vi "Set ADC.vi"(8 "error in (no error)":errorcluster, 10 "Configure ADS1115":T1={"Mode"=enum."Single-Shot", "MUX"=enum."Single AI3 - GND", "Data Rate"=enum."8 SPS", "PGA"=enum."FS = ±6.144V"}, 11 "ADS1115 in":refnum<class "Grove An In ADS1115.lvclass">) -> (0 "error out":errorcluster, 3 "ADS1115 out":refnum<class "Grove An In ADS1115.lvclass">)   [LabVIEW 2020, in "CTI-Peripheral.lvlib" / "Grove An In ADS1115.lvclass"]
uses:
  Grove An In ADS1115.lvclass
  Private/ConfigData.ctl
  Private/ADS1115Mode.ctl
  Private/ADS1115Mux.ctl
  Private/ADS1115DataRate.ctl
  Private/ADS1115PGA.ctl
  Grove An In ADS1115.lvclass/Grove An In ADS1115.ctl
  CTI/I2C Connection/I2C Connection.lvclass/I2C Connection.ctl
  CTI/Session/I2C Write Data.vi
  CTI/Session/I2C Read Data.vi
  CTI/I2C Connection/I2C Connection.lvclass
panel:
  out "Data":string
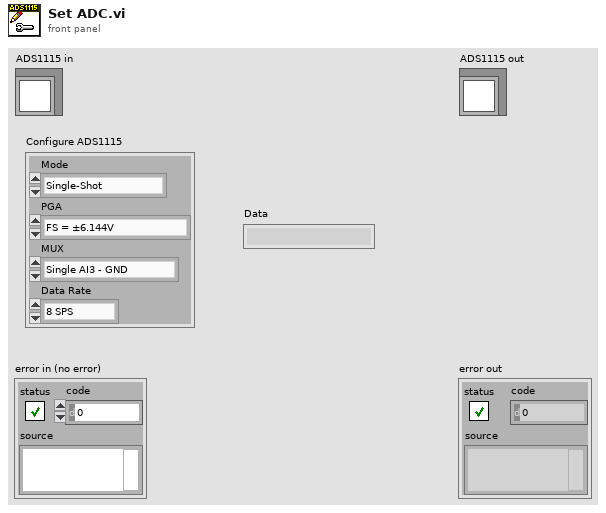
[diagram p1: front panel]
types:
  T1 = typedef "ConfigData.ctl" = cluster{"Mode":T2, "MUX":T3, "Data Rate":T4, "PGA":T5}
  T2 = typedef "CTI-Peripheral.lvlib/Grove An In ADS1115.lvclass/ADS1115Mode.ctl" = enum16{"Continuous", "Single-Shot"}
  T3 = typedef "CTI-Peripheral.lvlib/Grove An In ADS1115.lvclass/ADS1115Mux.ctl" = enum16{"Single AI0 - GND", "Single AI1 - GND", "Single AI2 - GND", "Single AI3 - GND"}
  T4 = typedef "CTI-Peripheral.lvlib/Grove An In ADS1115.lvclass/ADS1115DataRate.ctl" = enum16{"8 SPS", "16 SPS", "32 SPS", "64 SPS", "128 SPS", "250 SPS", "475 SPS", "860 SPS"}
  T5 = typedef "CTI-Peripheral.lvlib/Grove An In ADS1115.lvclass/ADS1115PGA.ctl" = enum16{"FS = ±6.144V", "FS = ±4.096V", "FS = ±2.048V", "FS = ±1.024V", "FS = ±0.512V", "FS = ±0.256V"}
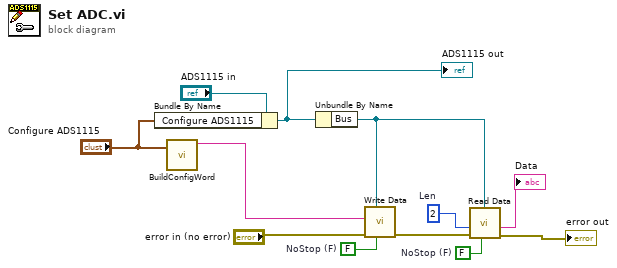
[diagram p0: block diagram]
diagram:
  w9 = FALSE  # NoStop (F)
  w10 = u8 2  # Len
  w11 = FALSE  # NoStop (F)
  n1 = Bundle By Name(cluster="ADS1115 in", "Configure ADS1115"="Configure ADS1115") -> (w1:refnum<class "Grove An In ADS1115.lvclass">)
  "ADS1115 out" <- w1
  n2 = call "BuildConfigWord.vi"("NewVal"="Configure ADS1115") -> ("string"=w5:string)  [unwired: 10 in]
  n3 = Unbundle By Name(w1) -> ("Bus"=w8:refnum<class "I2C Connection.lvclass">)
  n4 = call "Write Data.vi"("NoStop (F)"=w11, "I2C Connection"=w8, "error in (no error)"="error in (no error)", "Data"=w5) -> ("error out"=w7:errorcluster)  [unwired: 7 in]
  n5 = call "Read Data.vi"("NoStop (F)"=w9, "I2C Connection"=w8, "error in (no error)"=w7, "Len"=w10) -> ("error out"=→"error out":errorcluster, "Data"=→"Data":string)  [unwired: 6 in]
